vi "NotifyIcon - Create ContextMenu.vi"(8 "error in":errorcluster, 11 "Menus":string[][](array[string])) -> (0 "error out":errorcluster, 3 "ContextMenu reference":refnum<k24>)   [LabVIEW 2018]
uses:
  System.Windows.Forms
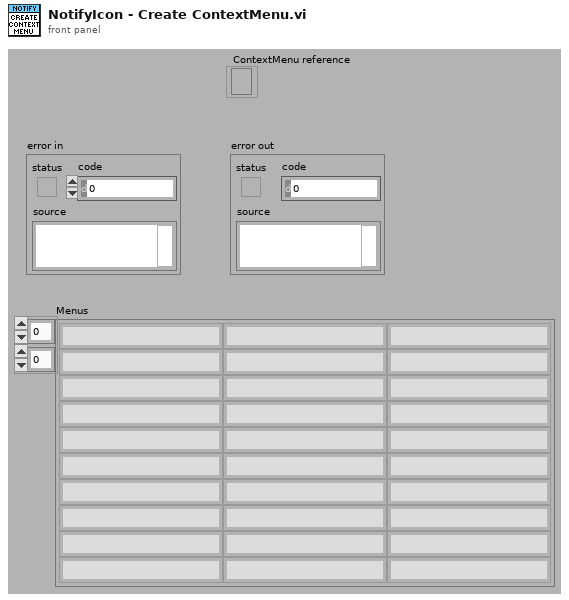
[diagram p1: front panel]
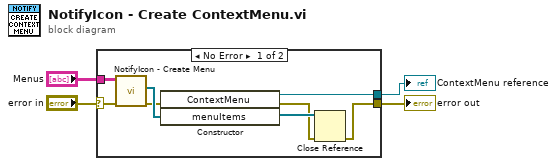
[diagram p0: block diagram]
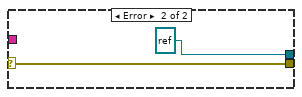
[diagram p2: hidden frame]
diagram:
  n1 = case shown="No Error" "error in" {
    selector: "error in" -> [w8 w14]
    tunnel: [w5 w14] -> w4
    tunnel: [w10 refnum<k24> refnum ("new reference")] -> w3
    tunnel: "Menus" -> [w9 _]
    frame No Error {
      n2 = call "NotifyIcon - Create Menu.vi"("error in"=w8, "Menus"=w9) -> ("error out"=w11:errorcluster, "MenuItem references"=w12:refnum<k24>[])  [unwired: 8 in]
      n3 = constructor class="ContextMenu"(error in=w11, "menuItems"=w12) -> (reference out=w10:refnum<k24>, error out=w6:errorcluster, "menuItems"=w7:refnum<k24>[])  [unwired: 2 in, 1 out]
      n4 = Close Reference(reference=w7, error in (no error)=w6) -> (error out=w5:errorcluster)
    }
    frame Error {
    }
  }
  "error out" <- w4
  "ContextMenu reference" <- w3
